vi "Add or Remove NULL from List.vi"(8 "error in (no error)":errorcluster, 10 "Add NULL Value":bool, 11 "List Data Type in":refnum<class "List Data Type.lvclass">) -> (0 "error out":errorcluster, 3 "List Data Type out":refnum<class "List Data Type.lvclass">)   [LabVIEW 2018, in "List Data Type.lvclass"]
uses:
  List Data Type.lvclass
  List Data Type.lvclass/List Data Type.ctl
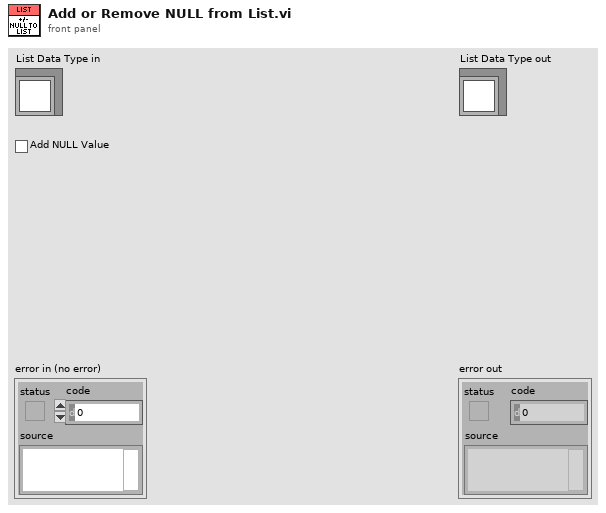
[diagram p1: front panel]
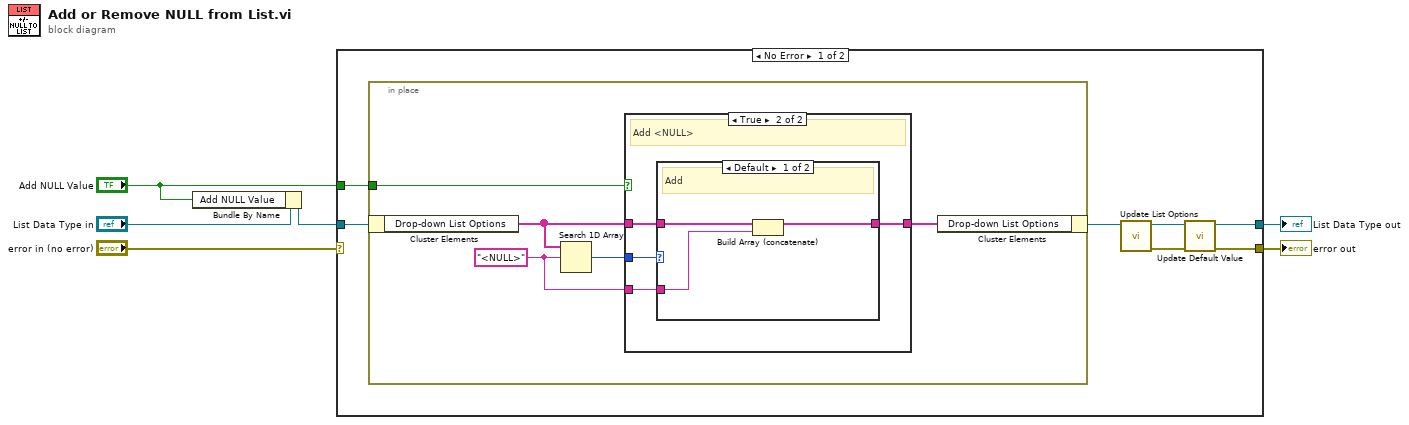
[diagram p0: block diagram]
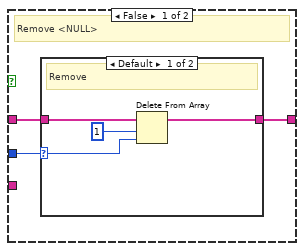
[diagram p2: hidden frame]
diagram:
  n1 = Bundle By Name(cluster="List Data Type in", "Add NULL Value"="Add NULL Value") -> (w2:refnum<class "List Data Type.lvclass">)
  n2 = case shown="No Error" "error in (no error)" {
    selector: "error in (no error)" -> [_ w36]
    tunnel: [w7 w36] -> w5
    tunnel: [w9 w35] -> w4
    tunnel: w2 -> [w13 w35]
    tunnel: "Add NULL Value" -> [w12 _]
    frame No Error {
      n3 = in-place {
        in-place-border: w12 -> [w18]
        w14 = "<NULL>" ("element")
        n4 = in-place-cluster #1(w13) -> ("Drop-down List Options"=w17:string[])
        n5 = Search 1D Array(1D array=w17, element=w14) -> (index of element=w16:i32)  [unwired: 1 in]
        n6 = case shown="True" w18 {
          tunnel: w17 -> [w19 w28]
          tunnel: w16 -> [w21 w30]
          tunnel: [w20 w29] -> w15
          tunnel: w14 -> [_ w27]
          frame False {
            # "Remove <NULL>"
            n7 = case shown="Default" w21 {
              selector: w21 -> [w22 _]
              tunnel: [w24 w26] -> w20
              tunnel: w19 -> [w25 w26]
              frame Default {
                # "Remove"
                n8 = Delete From Array(array=w25, length=1, index=w22) -> (array with subset deleted=w24:string[])  [unwired: 1 out]
              }
              frame -1 {
                # "Does Not Exist.  Doo Nothing."
              }
            }
          }
          frame True {
            # "Add <NULL>"
            n9 = case shown="Default" w30 {
              tunnel: [w31 w34] -> w29
              tunnel: w28 -> [w33 w34]
              tunnel: w27 -> [w32 _]
              frame Default {
                # "Add"
                n10 = Build Array (concatenate)(w33, w32) -> (w31:string[])
              }
              frame 0.. {
                # "Already Exists. Do Nothing."
              }
            }
          }
        }
        n11 = in-place-cluster #1("Drop-down List Options"=w15) -> (w11:refnum<class "List Data Type.lvclass">)
      }
      n12 = call "Update List Options.vi"("List Data Type in"=w11) -> ("error out"=w8:errorcluster, "List Data Type out"=w10:refnum<class "List Data Type.lvclass">)  [unwired: 9 in]
      n13 = call "Update Default Value.vi"("error in (no error)"=w8, "List Data Type in"=w10) -> ("error out"=w7:errorcluster, "List Data Type out"=w9:refnum<class "List Data Type.lvclass">)  [unwired: 8 in]
    }
    frame Error {
    }
  }
  "error out" <- w5
  "List Data Type out" <- w4
